vi "write to database.vi"(4 "2D data":string[][](array[string]) caption="2D Data", 6 "data in":string[](array[string]) caption="1D Data", 7 "Header":string[](array[string]), 8 "error in (no error)":errorcluster caption="错误输入（无错误）", 10 "file name":string, 11 "path":path) -> (0 "error out":errorcluster caption="错误输出", 3 "new file path (Not A Path if cancelled)":path)   [LabVIEW 2018]
uses:
  <vilib>/Utility/file.llb/Write To Spreadsheet File (string).vi
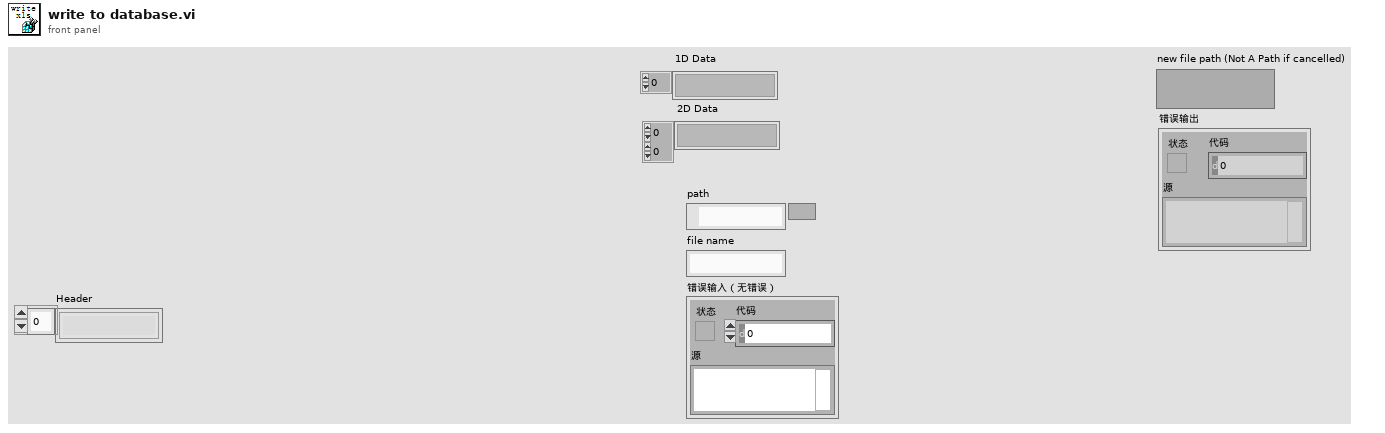
[diagram p1: front panel]
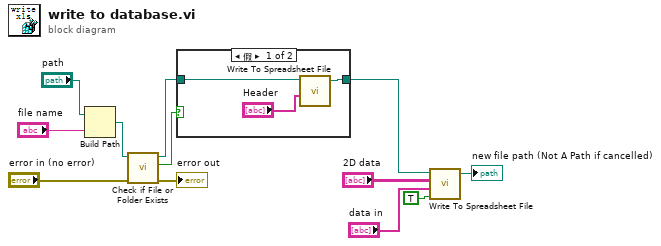
[diagram p0: block diagram]
diagram:
  n1 = Build Path(base path="path", name or relative path="file name") -> (appended path=w10:path)
  n2 = call <vilib>:"Check if File or Folder Exists.vi"("error in (no error)"="error in (no error)", "path"=w10) -> ("error out"=→"error out":errorcluster, "file or folder exists?"=w8:bool, "dup path"=w7:path)  [unwired: 7 in]
  n3 = case shown="假" w8 {
    tunnel: [w14 w16] -> w6
    tunnel: w7 -> [w15 w16]
    frame False {
      n4 = call-poly <vilib>:"Write To Spreadsheet File.vi"("1D data"="Header", "file path (dialog if empty)"=w15) -> ("new file path (Not A Path if cancelled)"=w14:path)  [unwired: 6 in]
    }
    frame True {
    }
  }
  n5 = call-poly <vilib>:"Write To Spreadsheet File.vi"("append to file? (new file:F)"=TRUE, "1D data"="data in", "2D data"="2D data", "file path (dialog if empty)"=w6) -> ("new file path (Not A Path if cancelled)"=→"new file path (Not A Path if cancelled)":path)  [unwired: 4 in]
